vi "Copy Template Files.vi"(8 "error in (no error)":errorcluster, 10 "Server Library (Library Item) in":refnum<vi>, 11 "Template Library (Library Item) in":refnum<vi>) -> (0 "error out":errorcluster, 2 "Server Library (Library Item) out":refnum<vi>, 3 "Template Library (Library Item) out":refnum<vi>)   [LabVIEW 2019, in "gRPC Scripting Tools.lvlib"]
uses:
  gRPC Scripting Tools.lvlib
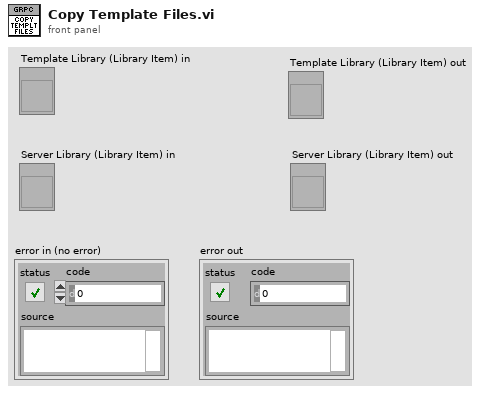
[diagram p1: front panel]
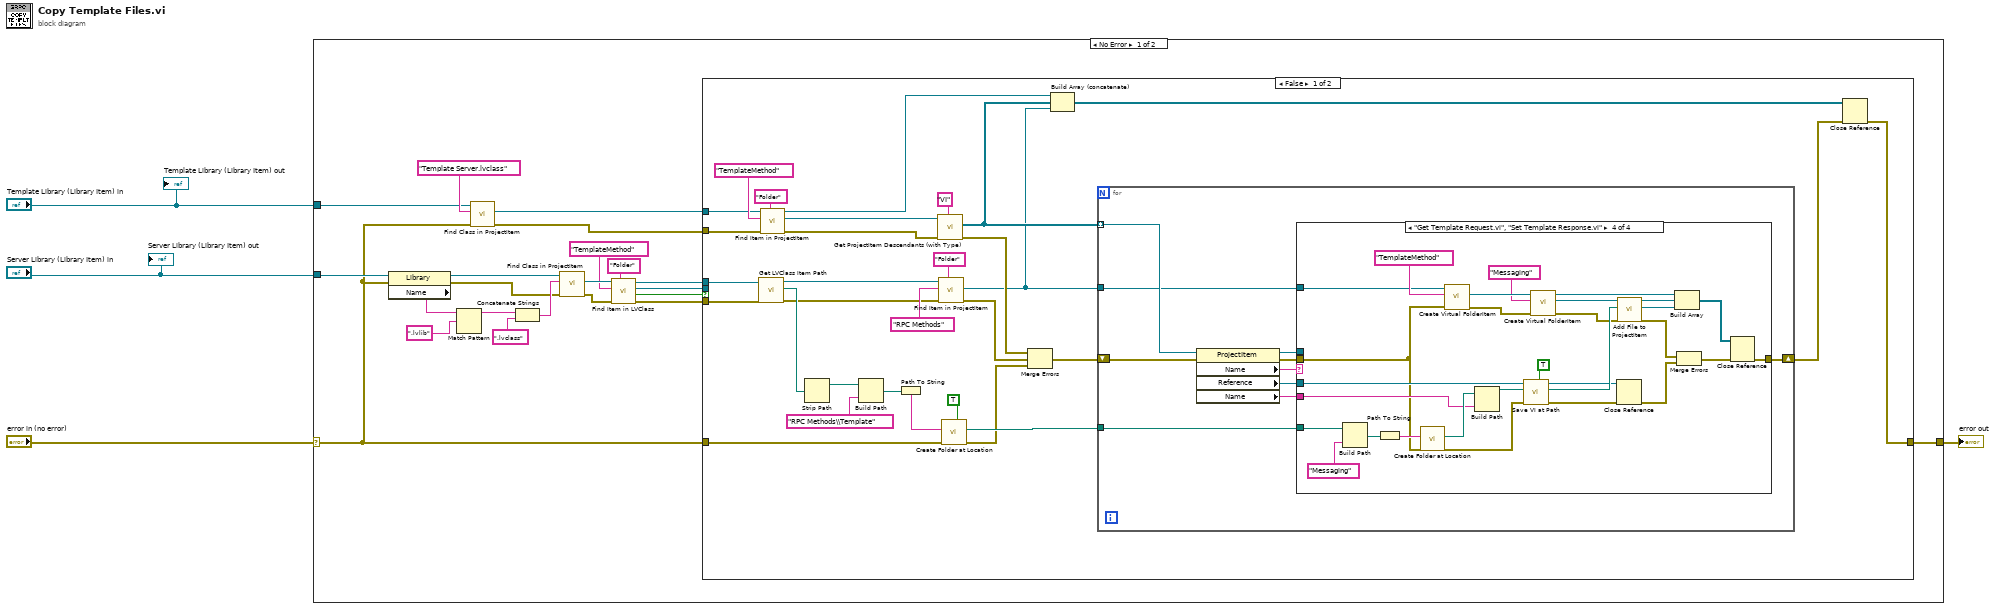
[diagram p0: block diagram]
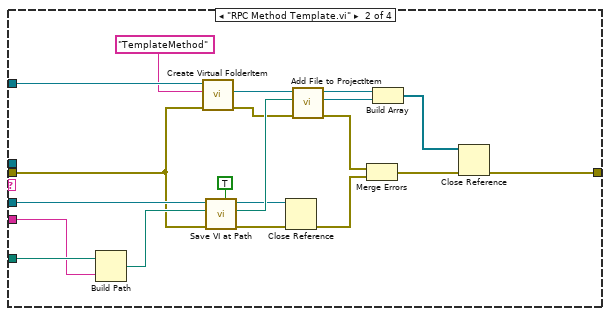
[diagram p3: hidden frame]
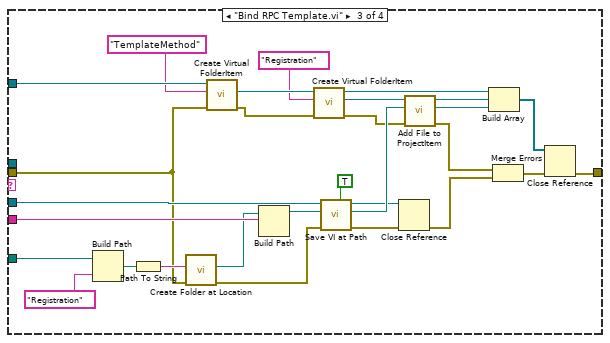
[diagram p4: hidden frame]
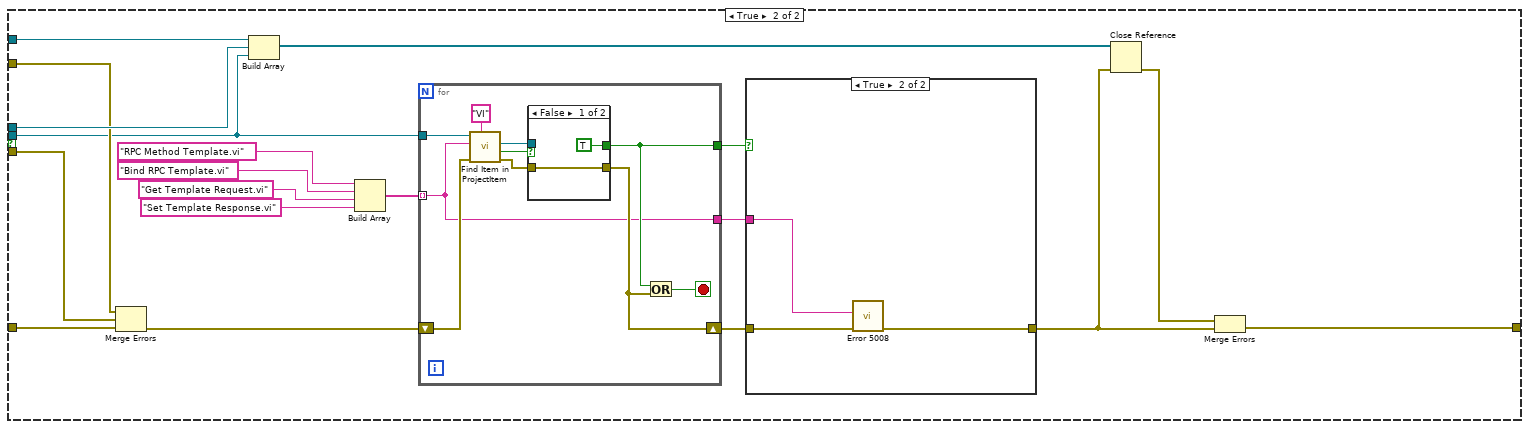
[diagram p5: hidden frame]
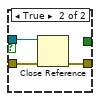
[diagram p7: hidden frame]
diagram:
  n1 = case shown="No Error" "error in (no error)" {
    selector: "error in (no error)" -> [w15 w184]
    tunnel: "Template Library (Library Item) in" -> [w25 _]
    tunnel: "Server Library (Library Item) in" -> [w23 _]
    tunnel: [w13 w184] -> w1
    frame No Error {
      n2 = property class="Library"(reference=w23, error in=w15) -> (reference out=w18:refnum<vi>, error out=w16:errorcluster, "Name"=w22:string)
      n3 = Match Pattern(string=w22, regular expression=".lvlib") -> (before substring=w20:string)  [unwired: 1 in, 3 out]
      n4 = call "Find Class in ProjectItem.vi"("error in (no error)"=w15, "Class Name"="Template Server.lvclass", "ProjectItem in"=w25) -> ("error out"=w14:errorcluster, "LVClass out"=w24:refnum<vi>)  [unwired: 5 in, 2 out]
      n5 = Concatenate Strings(w20, ".lvclass" ("string")) -> (w17:string)
      n6 = call "Find Class in ProjectItem.vi"("error in (no error)"=w16, "Class Name"=w17, "ProjectItem in"=w18) -> ("error out"=w12:errorcluster, "LVClass out"=w10:refnum<vi>)  [unwired: 5 in, 2 out]
      n7 = call "Find Item in LVClass.vi"("Item Type"="Folder", "error in (no error)"=w12, "Item Name"="TemplateMethod" ("Name"), "Class Item in"=w10) -> ("error out"=w6:errorcluster, "Found?"=w8:bool, "Project Item (Class Item)"=w5:refnum<vi>, "Class Item out"=w7:refnum<vi>)  [unwired: 4 in]
      n8 = case shown="False" w8 {
        tunnel: w24 -> [w55 w164]
        tunnel: w15 -> [w44 w162]
        tunnel: w14 -> [w43 w160]
        tunnel: [w32 w148] -> w13
        tunnel: w6 -> [w27 w161]
        tunnel: w7 -> [w28 w163]
        tunnel: w5 -> [_ w158]
        frame False {
          n9 = call "Get LVClass Item Path.vi"("error in (no error)"=w27, "LVClassLibrary in"=w28) -> ("error out"=w29:errorcluster, "Path"=w31:path, "LVClassLibrary out"=w30:refnum<vi>)  [unwired: 7 in]
          n10 = call "Find Item in ProjectItem.vi"("Item Type"="Folder", "error in (no error)"=w43, "Name"="TemplateMethod", "ProjectItem in"=w55) -> ("error out"=w42:errorcluster, "Item Refnum out"=w54:refnum<vi>, "ProjectItem out"=w37:refnum<vi>)  [unwired: 4 in, 1 out]
          n11 = Strip Path(path=w31) -> (stripped path=w52:path)  [unwired: 1 out]
          n12 = Build Path(base path=w52, name or relative path="RPC Methods\\Template") -> (appended path=w49:path)
          n13 = Path To String(path=w49) -> (string=w48:string)
          n14 = call "Get ProjectItem Descendants (with Type).vi"("Type"="VI", "error in (no error)"=w42, "ProjectItem in"=w54) -> ("error out"=w40:errorcluster, "All Descendents"=w36:refnum<vi>[])  [unwired: 6 in, 1 out]
          n15 = call "Find Item in ProjectItem.vi"("Item Type"="Folder", "error in (no error)"=w29, "Name"="RPC Methods", "ProjectItem in"=w30) -> ("error out"=w39:errorcluster, "Item Refnum out"=w35:refnum<vi>)  [unwired: 4 in, 2 out]
          n16 = call "Create Folder at Location.vi"("Override existing (F)"=TRUE, "Error In"=w44, "Path"=w48) -> ("Error Out"=w41:errorcluster, "Full path out"=w47:path)  [unwired: 6 in, 1 out]
          n17 = Merge Errors(w40, w39, w41) -> (w38:errorcluster)
          n18 = Build Array (concatenate)(w37, w36, w35) -> (w34:refnum<vi>[])
          n19 = for {
            tunnel: w36 -> [w67] mode=indexing
            tunnel: w47 -> [w64]
            tunnel: w35 -> [w62]
            shift-right: [w58] -> w33
            shift-left: w38 -> [w60]
            n20 = property class="ProjectItem"(reference=w67, error in=w60) -> (reference out=w65:refnum<vi>, error out=w59:errorcluster, "Name"=w66:string, "Reference"=w61:refnum<vi>, "Name"=w63:string)
            n21 = case shown="\"Get Template Request.vi\", \"Set Template Response.vi\"" w66 {
              tunnel: w65 -> [_ _ _ _]
              tunnel: w64 -> [_ w88 w114 w145]
              tunnel: w63 -> [_ w87 w117 w140]
              tunnel: w62 -> [_ w86 w107 w135]
              tunnel: w61 -> [_ w82 w112 w138]
              tunnel: w59 -> [w68 w79 w103 w131]
              tunnel: [w68 w72 w92 w121] -> w58
              frame "None", Default {
              }
              frame "RPC Method Template.vi" {
                n22 = Build Path(base path=w88, name or relative path=w87) -> (appended path=w81:path)
                n23 = call "Create Virtual FolderItem.vi"("error in (no error)"=w79, "Folder Name"="TemplateMethod", "ProjectItem in"=w86) -> ("error out"=w78:errorcluster, "FolderItem reference out"=w84:refnum<vi>)  [unwired: 5 in, 2 out]
                n24 = call "Save VI at Path.vi"("Save a Copy (F)"=TRUE, "error in (no error)"=w79, "Path"=w81, "VI in"=w82) -> ("error out"=w71:errorcluster, "Path to saved File"=w80:path, "VI out"=w70:refnum<vi>)  [unwired: 5 in]
                n25 = Close Reference(reference=w70, error in (no error)=w71) -> (error out=w69:errorcluster)
                n26 = call "Add File to ProjectItem.vi"("error in (no error)"=w78, "File Path"=w80, "ProjectItem in"=w84) -> ("error out"=w77:errorcluster, "Added File ref"=w75:refnum<vi>, "ProjectItem out"=w76:refnum<vi>)  [unwired: 6 in]
                n27 = Merge Errors(w77, w69) -> (w74:errorcluster)
                n28 = Build Array(w76, w75) -> (w73:refnum<vi>[])
                n29 = Close Reference(reference=w73, error in (no error)=w74) -> (error out=w72:errorcluster)
              }
              frame "Bind RPC Template.vi" {
                n30 = Build Path(base path=w114, name or relative path="Registration") -> (appended path=w116:path)
                n31 = Path To String(path=w116) -> (string=w115:string)
                n32 = call "Create Folder at Location.vi"("Error In"=w103, "Path"=w115) -> ("Error Out"=w100:errorcluster, "Full path out"=w99:path)  [unwired: 7 in, 1 out]
                n33 = call "Create Virtual FolderItem.vi"("error in (no error)"=w103, "Folder Name"="TemplateMethod", "ProjectItem in"=w107) -> ("error out"=w102:errorcluster, "FolderItem reference out"=w109:refnum<vi>)  [unwired: 5 in, 2 out]
                n34 = Build Path(base path=w99, name or relative path=w117) -> (appended path=w110:path)
                n35 = call "Create Virtual FolderItem.vi"("error in (no error)"=w102, "Folder Name"="Registration", "ProjectItem in"=w109) -> ("error out"=w101:errorcluster, "FolderItem reference out"=w104:refnum<vi>, "ProjectItem out"=w96:refnum<vi>)  [unwired: 5 in, 1 out]
                n36 = call "Save VI at Path.vi"("Save a Copy (F)"=TRUE, "error in (no error)"=w100, "Path"=w110, "VI in"=w112) -> ("error out"=w91:errorcluster, "Path to saved File"=w105:path, "VI out"=w90:refnum<vi>)  [unwired: 5 in]
                n37 = Close Reference(reference=w90, error in (no error)=w91) -> (error out=w89:errorcluster)
                n38 = call "Add File to ProjectItem.vi"("error in (no error)"=w101, "File Path"=w105, "ProjectItem in"=w104) -> ("error out"=w98:errorcluster, "Added File ref"=w94:refnum<vi>, "ProjectItem out"=w95:refnum<vi>)  [unwired: 6 in]
                n39 = Build Array(w96, w95, w94) -> (w93:refnum<vi>[])
                n40 = Merge Errors(w98, w89) -> (w97:errorcluster)
                n41 = Close Reference(reference=w93, error in (no error)=w97) -> (error out=w92:errorcluster)
              }
              frame "Get Template Request.vi", "Set Template Response.vi" {
                n42 = Build Path(base path=w145, name or relative path="Messaging") -> (appended path=w143:path)
                n43 = Path To String(path=w143) -> (string=w142:string)
                n44 = call "Create Folder at Location.vi"("Error In"=w131, "Path"=w142) -> ("Error Out"=w130:errorcluster, "Full path out"=w141:path)  [unwired: 7 in, 1 out]
                n45 = call "Create Virtual FolderItem.vi"("error in (no error)"=w131, "Folder Name"="TemplateMethod", "ProjectItem in"=w135) -> ("error out"=w129:errorcluster, "FolderItem reference out"=w134:refnum<vi>)  [unwired: 5 in, 2 out]
                n46 = Build Path(base path=w141, name or relative path=w140) -> (appended path=w137:path)
                n47 = call "Save VI at Path.vi"("Save a Copy (F)"=TRUE, "error in (no error)"=w130, "Path"=w137, "VI in"=w138) -> ("error out"=w120:errorcluster, "Path to saved File"=w132:path, "VI out"=w119:refnum<vi>)  [unwired: 5 in]
                n48 = call "Create Virtual FolderItem.vi"("error in (no error)"=w129, "Folder Name"="Messaging", "ProjectItem in"=w134) -> ("error out"=w128:errorcluster, "FolderItem reference out"=w125:refnum<vi>, "ProjectItem out"=w126:refnum<vi>)  [unwired: 5 in, 1 out]
                n49 = Close Reference(reference=w119, error in (no error)=w120) -> (error out=w118:errorcluster)
                n50 = call "Add File to ProjectItem.vi"("error in (no error)"=w128, "File Path"=w132, "ProjectItem in"=w125) -> ("error out"=w127:errorcluster, "Added File ref"=w124:refnum<vi>)  [unwired: 6 in, 1 out]
                n51 = Build Array(w126, w125, w124) -> (w122:refnum<vi>[])
                n52 = Merge Errors(w127, w118) -> (w123:errorcluster)
                n53 = Close Reference(reference=w122, error in (no error)=w123) -> (error out=w121:errorcluster)
              }
            }
          }
          n54 = Close Reference(reference=w34, error in (no error)=w33) -> (error out=w32:errorcluster)
        }
        frame True {
          n55 = Merge Errors(w160, w161, w162) -> (w152:errorcluster)
          n56 = Build Array(w164, w163, w158) -> (w159:refnum<vi>[])
          n57 = Build Array("RPC Method Template.vi" ("Name"), "Bind RPC Template.vi" ("element"), "Get Template Request.vi" ("element"), "Set Template Response.vi" ("element")) -> (w153:string[])
          n58 = for {
            tunnel: w158 -> [w178]
            tunnel: w153 -> [w169] mode=indexing
            shift-right: [w171] -> w151
            shift-left: w152 -> [w174]
            tunnel: [w170] -> w150
            tunnel: [w169] -> w149
            stop <- w172 stop-if-true
            n59 = call "Find Item in ProjectItem.vi"("Item Type"="VI", "error in (no error)"=w174, "Name"=w169, "ProjectItem in"=w178) -> ("error out"=w173:errorcluster, "Found ?"=w176:bool, "Item Refnum out"=w175:refnum<vi>)  [unwired: 4 in, 1 out]
            n60 = case shown="False" w176 {
              tunnel: w175 -> [_ w183]
              tunnel: w173 -> [w180 w182]
              tunnel: [w180 w181] -> w171
              tunnel: [TRUE _] -> w170
              frame False {
              }
              frame True {
                n61 = Close Reference(reference=w183, error in (no error)=w182) -> (error out=w181:errorcluster)
              }
            }
            n62 = Or(x=w170, y=w171) -> (x .or. y?=w172:bool)
          }
          n63 = case shown="True" w150 {
            tunnel: w151 -> [w165 w168]
            tunnel: w149 -> [_ w167]
            tunnel: [w165 w166] -> w146
            frame False {
            }
            frame True {
              n64 = call "Error 5008.vi"("error in (no error)"=w168, "File Name"=w167) -> ("error out"=w166:errorcluster)  [unwired: 9 in]
            }
          }
          n65 = Close Reference(reference=w159, error in (no error)=w146) -> (error out=w147:errorcluster)
          n66 = Merge Errors(w147, w146) -> (w148:errorcluster)
        }
      }
    }
    frame Error {
    }
  }
  "error out" <- w1
  "Template Library (Library Item) out" <- "Template Library (Library Item) in"
  "Server Library (Library Item) out" <- "Server Library (Library Item) in"
